vi "host - network - RT (separate).vi"() -> (1 "Fx":dbl, 2 "Tz":dbl, 3 "Fy":dbl, 4 "Fz":dbl, 5 "Tx":dbl, 6 "Ty":dbl)   [LabVIEW 2010]
uses:
  <vilib>/Analysis/Matrix/NI_Matrix.lvlib
  <vilib>/Analysis/Matrix/Numeric/Multiply/Multiply - RM,RM.vi
  <vilib>/Analysis/Matrix/Numeric/Conversions/Array To Matrix - RA2.vi
  <vilib>/Analysis/Matrix/Numeric/Conversions/Array To Matrix - RA.vi
  <vilib>/Analysis/Matrix/Numeric/Conversions/Matrix To Array - RM.vi
panel:
  in  "Reset logging":bool
  out "appended path":path
  out "Bias Vector":dbl[](array[numeric])
  out "Scale Matrix":dbl[][](array[numeric])=[[1.0, 0.0, 0.0, 0.0, 0.0, 0.0], [0.0, 1.0, 0.0, 0.0, 0.0, 0.0], [0.0, 0.0, 1.0, 0.0, 0.0, 0.0], [0.0, 0.0, 0.0, 1.0, 0.0, 0.0], [0.0, 0.0, 0.0, 0.0, 1.0, 0.0], [0.0, 0.0, 0.0, 0.0, 0.0, 1.0]]
  out "Analog Inputs":dbl[](array[numeric])
  out "Temp":dbl(graph)
  out "Tz":dbl(graph)
  out "Ty":dbl(graph)
  out "Tx":dbl(graph)
  out "Fz":dbl(graph)
  out "Fy":dbl(graph)
  in  "stop":bool
  out "Fx":dbl(graph)
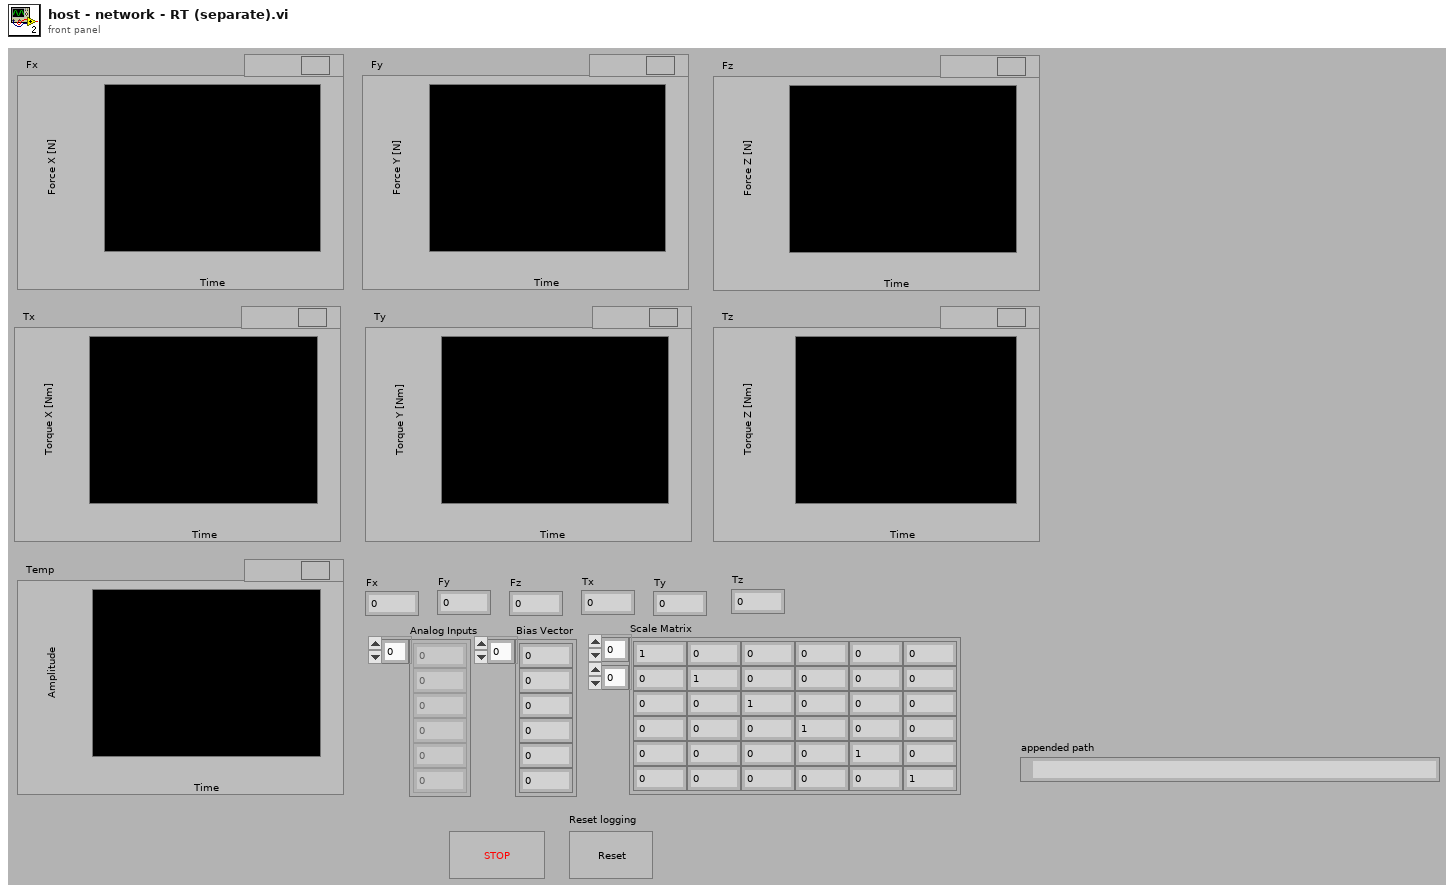
[diagram p1: front panel]
types:
  T1 = typedef "NI_Matrix.lvlib/RealMatrix.ctl" = dbl[][]
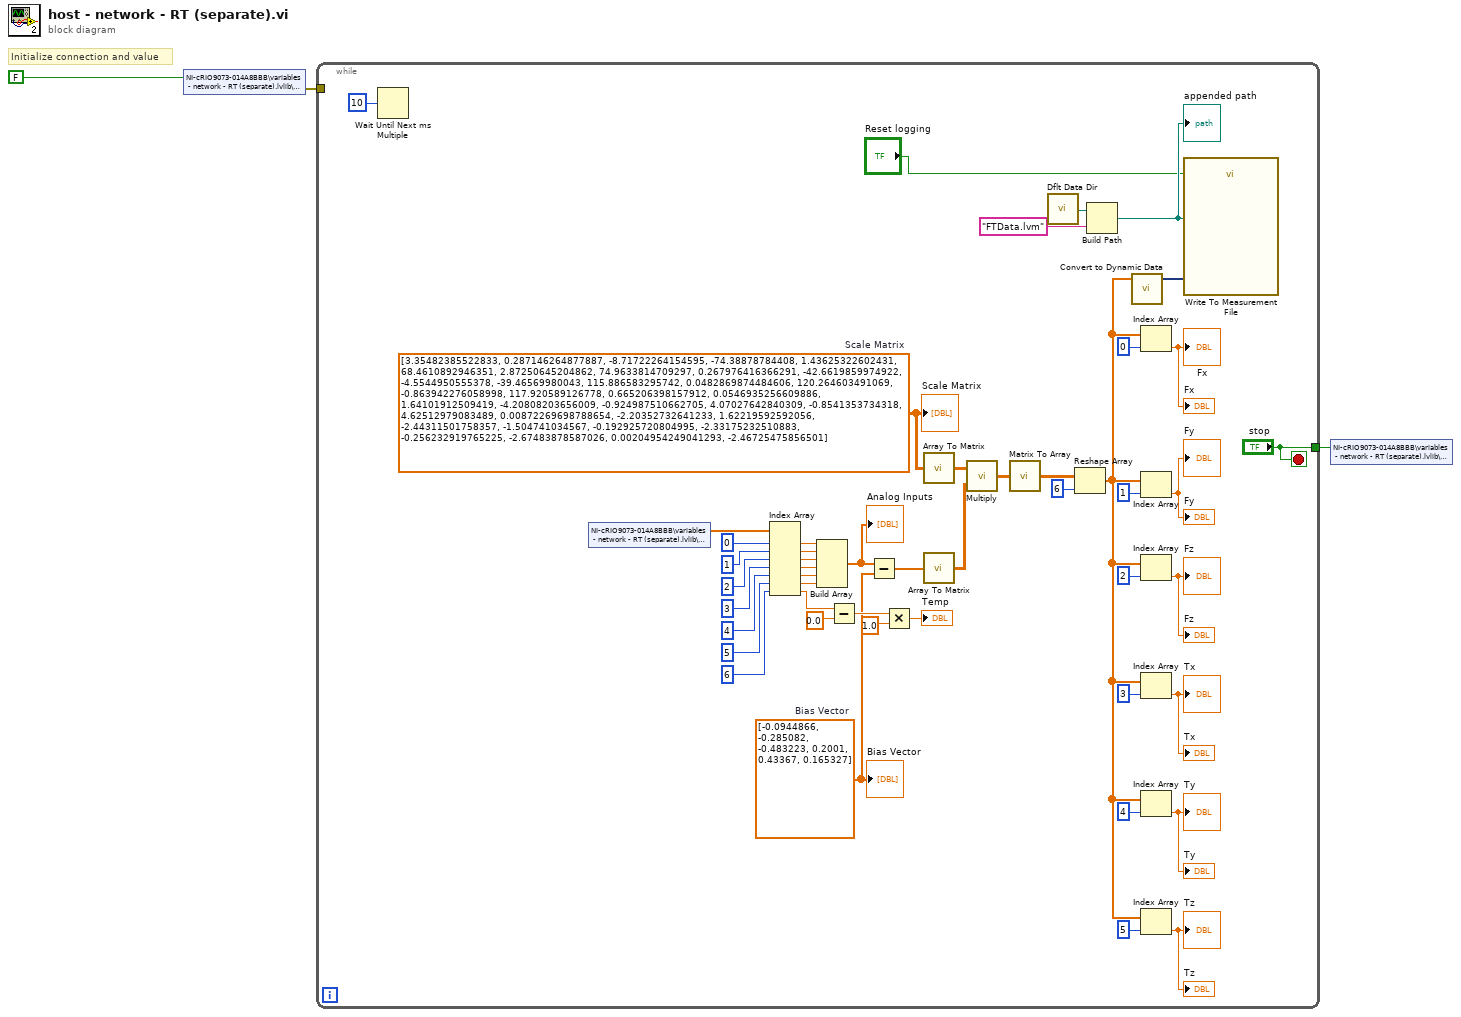
[diagram p0: block diagram]
diagram:
  # "Initialize connection and value"
  n1 = shared-variable "NI-cRIO9073-014A8BBB\\variables - network - RT (separate).lvlib\\stop - network"(FALSE) -> (error out=w2:errorcluster)  [unwired: 1 in]
  n2 = while {
    tunnel: ["stop"] -> w3
    tunnel: w2 -> [_]
    stop <- "stop" stop-if-true
    w23 = dbl[][] [[3.35482385522833, 0.287146264877887, -8.71722264154595, -74.38878784408, 1.43625322602431, 68.4610892946351], [2.87250645204862, 74.9633814709297, 0.267976416366291, -42.6619859974922, -4.5544950555378, -39.46569980043], [115.886583295742, 0.0482869874484606, 120.264603491069, -0.863942276058998, 117.920589126778, 0.665206398157912], [0.0546935256609886, 1.64101912509419, -4.20808203656009, -0.924987510662705, 4.07027642840309, -0.8541353734318], [4.62512979083489, 0.00872269698788654, -2.20352732641233, 1.62219592592056, -2.44311501758357, -1.504741034567], [-0.192925720804995, -2.33175232510883, -0.256232919765225, -2.67483878587026, 0.00204954249041293, -2.46725475856501]]  # Scale Matrix
    w12 = dbl[] [-0.0944866, -0.285082, -0.483223, 0.2001, 0.43367, 0.165327]  # Bias Vector
    n3 = Wait Until Next ms Multiple(millisecond multiple=u32 10) -> ()  [unwired: 1 out]
    n4 = shared-variable "NI-cRIO9073-014A8BBB\\variables - network - RT (separate).lvlib\\data - network"() -> (w49:dbl[])  [unwired: 1 in, 1 out]
    n5 = Index Array(array=w49, index #1=u32 0 ("millisecond multiple"), index #2=u32 1 ("millisecond multiple"), index #3=u32 2 ("millisecond multiple"), index #4=u32 3 ("millisecond multiple"), index #5=u32 4 ("millisecond multiple"), index #6=u32 5 ("millisecond multiple"), index #7=u32 6 ("millisecond multiple")) -> (element #1=w39:dbl, element #2=w38:dbl, element #3=w37:dbl, element #4=w36:dbl, element #5=w35:dbl, element #6=w34:dbl, element #7=w13:dbl)
    n6 = Build Array(w39, w38, w37, w36, w35, w34) -> (w41:dbl[])
    "Analog Inputs" <- w41
    n7 = Subtract(x=w13, y=0.0) -> (x-y=w16:dbl)
    n8 = Subtract(x=w41, y=w12) -> (x-y=w40:dbl[])
    n9 = Multiply(x=w16, y=1.0) -> (x*y=→"Temp":dbl)
    n10 = call-poly <vilib>:"Array To Matrix.vi"("Real 2D Array"=w23) -> ("Real Matrix"=w26:T1)
    n11 = call-poly <vilib>:"Array To Matrix.vi"("Real 1D Array"=w40) -> ("Real Matrix (Column Vector)"=w25:T1)
    n12 = call-poly <vilib>:"Multiply.vi"("Real Matrix B"=w25, "Real Matrix A"=w26) -> ("A * B"=w24:T1)
    n13 = call-poly <vilib>:"Matrix To Array.vi"("Real Matrix"=w24) -> ("Real 2D Array"=w6:dbl[][])
    n14 = call <vilib>:"Dflt Data Dir.vi"() -> ("App:Default Data Directory"=w10:path)
    n15 = Reshape Array(w6, 6 ("disabled index (col)")) -> (w5:dbl[])
    n16 = Build Path(base path=w10, name or relative path="FTData.lvm") -> (appended path=w8:path)
    "appended path" <- w8
    n17 = call "Convert to Dynamic Data"("Array"=w5) -> ("Dynamic Data Type"=w9:dynamicdata)  [unwired: 3 in]
    n18 = Index Array(array=w5, index=0) -> (element=→"Fx" →"Fx":dbl)
    n19 = Index Array(array=w5, index=1) -> (element=→"Fy" →"Fy":dbl)
    n20 = Index Array(array=w5, index=2) -> (element=→"Fz" →"Fz":dbl)
    n21 = Index Array(array=w5, index=3) -> (element=→"Tx" →"Tx":dbl)
    n22 = Index Array(array=w5, index=4) -> (element=→"Ty" →"Ty":dbl)
    n23 = Index Array(array=w5, index=5) -> (element=→"Tz" →"Tz":dbl)
    n24 = call "Write To Measurement File"("Signals"=w9, "Reset"="Reset logging", "Filename"=w8) -> ()  [unwired: 14 in, 3 out]
    "Scale Matrix" <- w23
    "Bias Vector" <- w12
  }
  n25 = shared-variable "NI-cRIO9073-014A8BBB\\variables - network - RT (separate).lvlib\\stop - network"(w3) -> ()  [unwired: 1 in, 1 out]
